vi "Messwerte fuer Modus aufbereiten.vi"(11 "GasValue":sgl[](array[numeric])) -> (3 "GasValue":sgl[](array[numeric]))   [LabVIEW 2020, in "ABB-EL3000.lvlib" / "FID.lvlib"]
uses:
  FID.lvlib
  FID Kalibrierung/Aktion FID Allgemeindaten.ctl
  FID Kalibrierung/FID Kalibrierung.lvlib
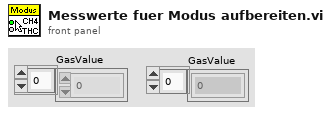
[diagram p1: front panel]
types:
  T1 = typedef "ABB-EL3000.lvlib/FID.lvlib/FID Kalibrierung.lvlib/Aktion FID Allgemeindaten.ctl" = enum16{"lesen", "Mod", "Time", "laden", "speichern"}
  T2 = typedef "ABB-EL3000.lvlib/FID.lvlib/Modus.ctl" = enum16{"Automatic", "CH4", "THC", "Efficienty measure", "Switching time"}
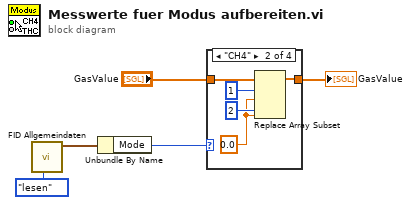
[diagram p0: block diagram]
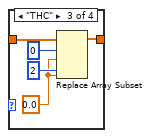
[diagram p3: hidden frame]
diagram:
  n1 = call "FID Allgemeindaten.vi"("Aktion"=Aktion_FID_Allgemeindaten."lesen") -> ("FID Allgemein"=w3:cluster{"Mode":T2, "Switching time":sgl})  [unwired: 9 in, 1 out]
  n2 = Unbundle By Name(w3) -> ("Mode"=w1:T2)
  n3 = case shown="\"CH4\"" w1 {
    tunnel: "GasValue" -> [w6 w11 w16 w17]
    tunnel: [w6 w7 w12 w17] -> w2
    frame "Automatic", Default {
    }
    frame "CH4" {
      w8 = sgl 0.0 ("Neues Element/Teil-Array")
      n4 = Replace Array Subset(array=w11, new element #1=w8, index #1=1 ("Index"), new element #2=w8, index #2=2 ("Index")) -> (w7:sgl[])
    }
    frame "THC" {
      w13 = sgl 0.0 ("Neues Element/Teil-Array")
      n5 = Replace Array Subset(array=w16, new element #1=w13, index #1=0 ("Index"), new element #2=w13, index #2=2 ("Index")) -> (w12:sgl[])
    }
    frame "Efficienty measure" {
    }
  }
  "GasValue" <- w2
